vi "FG Starting WP.vi"(1 "FG Action (Read)":T2, 2 "Starting WP in":T1 {"Longitude" format="%#_14g"; "Latitude" format="%#_14g"}) -> (0 "Starting WP out":T1 {"Longitude" format="%#_14g"; "Latitude" format="%#_14g"})   [LabVIEW 2009]
uses:
  Actions for FG's.ctl
  TypeDefs/Sensor TypeDefs/GPS Data.ctl
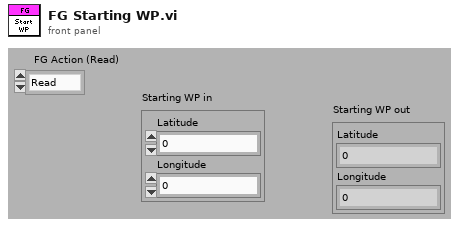
[diagram p1: front panel]
types:
  T1 = typedef "GPS Data.ctl" = cluster{"Latitude":dbl, "Longitude":dbl}
  T2 = typedef "Actions for FG's.ctl" = enum16{"Read", "Write"}
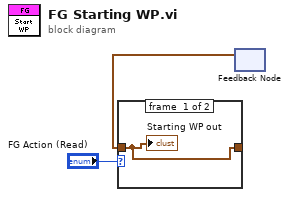
[diagram p0: block diagram]
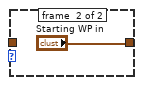
[diagram p2: hidden frame]
diagram:
  n1 = feedback #1() -> (w1:T1)  [unwired: 1 in]
  n2 = case shown="\"Read\", Default" "FG Action (Read)" {
    tunnel: [w4 "Starting WP in"] -> w2
    tunnel: w1 -> [w4 _]
    frame #0 {
      "Starting WP out" <- w4
    }
    frame #1 {
    }
  }
